vi "write_log_metadata.vi"(8 "error in (no error)":errorcluster, 10 "data":variant, 11 "raw_stream_logger in":refnum<class "raw_stream_logger.lvclass">) -> (0 "error out":errorcluster, 3 "raw_stream_logger out":refnum<class "raw_stream_logger.lvclass">)   [LabVIEW 2015, in "raw_stream_logger.lvclass"]
uses:
  raw_stream_logger.lvclass
  hdf5_photon_record_logger/stream_metadata.ctl
  hydraharp_panel/hpanel_hydraharp_settings.ctl
  hydraharp_panel/hpanel_sync_settings.ctl
  hydraharp_panel/hpanel_sync_div.ctl
  hydraharp_panel/hpanel_channel_settings.ctl
  Picoharp/picoharp/picoharp.lvclass
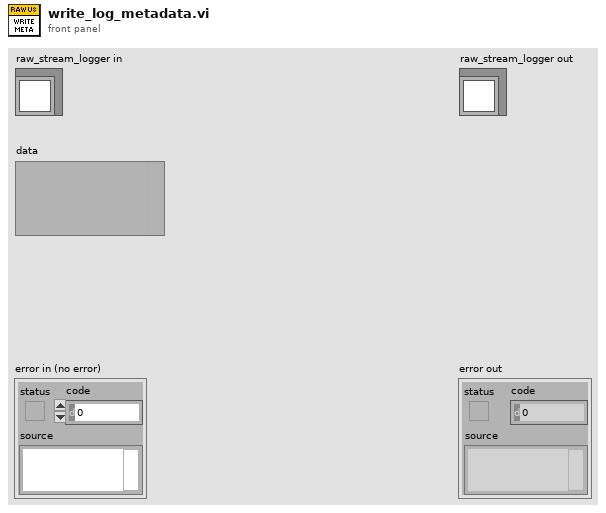
[diagram p1: front panel]
types:
  T1 = typedef "stream_metadata.ctl" = cluster{"Hydraharp Settings":T2, "resolution":dbl, "stream_notes":string}
  T2 = typedef "hpanel_hydraharp_settings.ctl" = cluster{"Sync Settings":T3, "CH 1":T5, "CH 2":T5, "CH 3":T5, "CH 4":T5, "binning":i32, "CH 5":T5, "CH 6":T5, "CH 7":T5, "CH 8":T5}
  T3 = typedef "hpanel_sync_settings.ctl" = cluster{"snc_count":i32, "snc_level":i32, "snc_ZeroX":i32, "snc_offs":i32, "sync_div":T4}
  T4 = typedef "hpanel_sync_div.ctl" = enum16{"1", "2", "4", "8"}
  T5 = typedef "hpanel_channel_settings.ctl" = cluster{"ch_counts":i32, "ch_level":i32, "ch_ZeroX":i32, "ch_offs":i32}
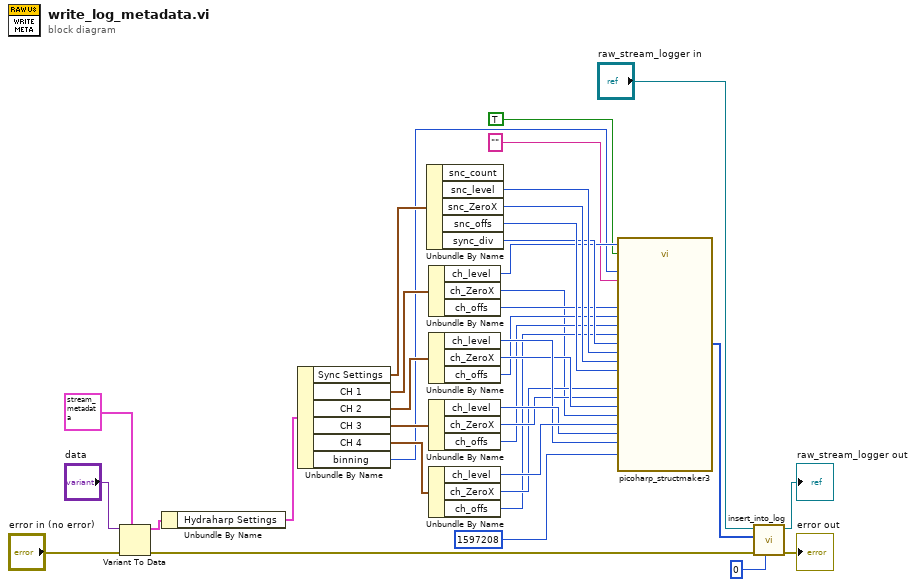
[diagram p0: block diagram]
diagram:
  n1 = Variant To Data(error in="error in (no error)", type=T1 {"Hydraharp Settings"={"Sync Settings"={"snc_count"=0, "snc_level"=0, "snc_ZeroX"=0, "snc_offs"=0, "sync_div"=enum."1"}, "CH 1"={"ch_counts"=0, "ch_level"=0, "ch_ZeroX"=0, "ch_offs"=0}, "CH 2"={"ch_counts"=0, "ch_level"=0, "ch_ZeroX"=0, "ch_offs"=0}, "CH 3"={"ch_counts"=0, "ch_level"=0, "ch_ZeroX"=0, "ch_offs"=0}, "CH 4"={"ch_counts"=0, "ch_level"=0, "ch_ZeroX"=0, "ch_offs"=0}, "binning"=0, "CH 5"={"ch_counts"=0, "ch_level"=0, "ch_ZeroX"=0, "ch_offs"=0}, "CH 6"={"ch_counts"=0, "ch_level"=0, "ch_ZeroX"=0, "ch_offs"=0}, "CH 7"={"ch_counts"=0, "ch_level"=0, "ch_ZeroX"=0, "ch_offs"=0}, "CH 8"={"ch_counts"=0, "ch_level"=0, "ch_ZeroX"=0, "ch_offs"=0}}, "resolution"=0.0, "stream_notes"="stream_notes"} ("output cluster"), Variant="data") -> (data=w6:T1, error out=w2:errorcluster)
  n2 = Unbundle By Name(w6) -> ("Hydraharp Settings"=w5:T2)
  n3 = Unbundle By Name(w5) -> ("Sync Settings"=w30:T3, "CH 1"=w28:T5, "CH 2"=w27:T5, "CH 3"=w26:T5, "CH 4"=w25:T5, "binning"=w8:i32)
  n4 = Unbundle By Name(w30) -> ("snc_level"=w17:i32, "snc_ZeroX"=w18:i32, "snc_offs"=w29:i32, "sync_div"=w16:T4)  [unwired: 1 out]
  n5 = Unbundle By Name(w28) -> ("ch_level"=w10:i32, "ch_ZeroX"=w11:i32, "ch_offs"=w12:i32)
  n6 = Unbundle By Name(w27) -> ("ch_level"=w22:i32, "ch_ZeroX"=w21:i32, "ch_offs"=w13:i32)
  n7 = Unbundle By Name(w26) -> ("ch_level"=w23:i32, "ch_ZeroX"=w20:i32, "ch_offs"=w14:i32)
  n8 = Unbundle By Name(w25) -> ("ch_level"=w24:i32, "ch_ZeroX"=w19:i32, "ch_offs"=w15:i32)
  n9 = call "picoharp_structmaker3.vi"("Channel 3 Zero Cross"=w19, "Channel 2 Zero Cross"=w20, "Channel 1 Zero Cross"=w21, "Channel 0 Zero Cross"=w11, "Channel 3 Discriminator"=w24, "Channel 2 Discriminator"=w23, "Channel 1 Discriminator"=w22, "Channel 0 Discriminator"=w10, "n_records"=1597208, "Use user inputs?"=TRUE, "Binning"=w8, "COMMENT"="", "Sync Offset"=w29, "Sync input Zero Cross Level"=w18, "Sync input Discriminator (mv)"=w17, "Sync Divider"=w16, "Channel 3 Offset"=w15, "Channel  2 Offset"=w14, "Channel 1 offset"=w13, "Channel 0 offset"=w12) -> ("Header in binary"=w4:u8[])  [unwired: 5 in, 2 out]
  n10 = call-dynamic "insert_into_log.vi"("offset_from_bof"=u32 0, "error in (no error)"=w2, "Data"=w4, "raw_stream_logger in"="raw_stream_logger in") -> ("error out"=→"error out":errorcluster, "raw_stream_logger out"=→"raw_stream_logger out":refnum<class "raw_stream_logger.lvclass">)  [unwired: 6 in]
